vi "SwitchStateControl.vi"(5 "Switch Bit":bool=TRUE, 8 "error in (no error)":errorcluster, 9 "IP":string="172.16.7.43", 11 "Port":u16=9764) -> (0 "error out":errorcluster)   [LabVIEW 2009]
panel:
  in  "N Bit":u16=10
  in  "Register Number":u16=4
  out "Register read swapped":u32=1078
  out "Register swap":dbl[](array[numeric])=[0.0, 1.0, 1.0, 0.0, 1.0, 1.0, 0.0, 0.0, 0.0, 0.0, 1.0, 0.0, 0.0, 0.0, 0.0, 0.0, 0.0, 0.0, 0.0, 0.0, 0.0, 0.0, 0.0, 0.0, 0.0, 0.0, 0.0, 0.0, 0.0, 0.0, 0.0, 0.0]
  out "Register 4 bits":dbl[](array[numeric])=[0.0, 1.0, 1.0, 0.0, 1.0, 1.0, 0.0, 0.0, 0.0, 0.0, 1.0, 0.0, 0.0, 0.0, 0.0, 0.0, 0.0, 0.0, 0.0, 0.0, 0.0, 0.0, 0.0, 0.0, 0.0, 0.0, 0.0, 0.0, 0.0, 0.0, 0.0, 0.0]
  out "Register read":u32=1078
  in  "Device":u16(ring)=4 items=["Attenuation", "Clipping", "Enable channel", "Delay line", "ASIC"]
  # "SumMaj Bit\n        ll\n        v"
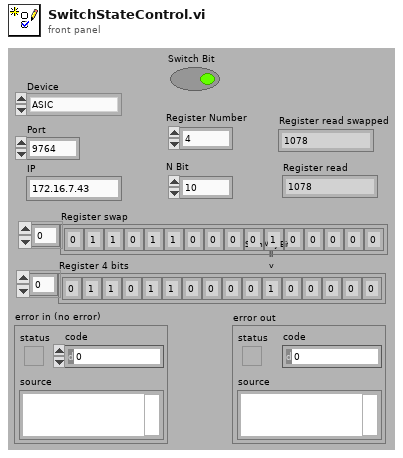
[diagram p1: front panel]
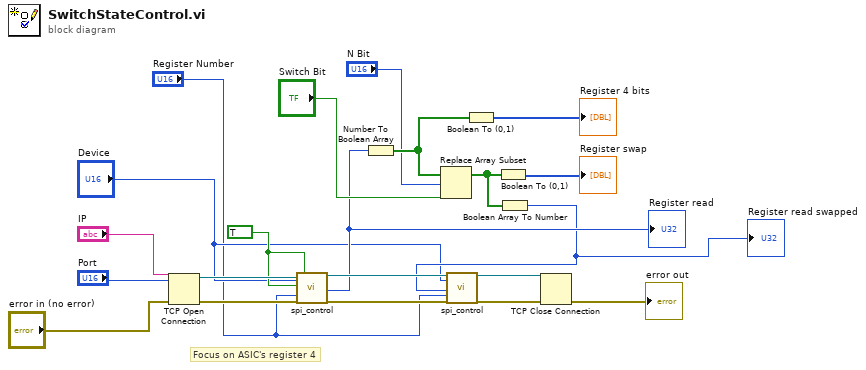
[diagram p0: block diagram]
diagram:
  w6 = TRUE
  # "Focus on ASIC's register 4"
  n1 = TCP Open Connection(address="IP", remote port or service name="Port", error in (no error)="error in (no error)") -> (connection ID=w18:refnum<k5>, error out=w19:errorcluster)  [unwired: 2 in]
  n2 = call "spi_control.vi"("connection ID"=w18, "Device"="Device", "Read/#write"=w6, "Register or channel"="Register Number", "error out 3"=w19, "Read physical"=w6) -> ("connection ID out"=w8:refnum<k5>, "data read value"=w5:u32, "error out 2"=w9:errorcluster)  [unwired: 6 in, 5 out]
  "Register read" <- w5
  n3 = Number To Boolean Array(number=w5) -> (Boolean array=w14:bool[])
  n4 = Replace Array Subset(array=w14, new element="Switch Bit", index="N Bit") -> (w11:bool[])
  n5 = Boolean To (0,1)(Boolean=w14) -> (0, 1=→"Register 4 bits":i16[])
  n6 = Boolean To (0,1)(Boolean=w11) -> (0, 1=→"Register swap":i16[])
  n7 = Boolean Array To Number(Boolean array=w11) -> (number=w4:u32)
  "Register read swapped" <- w4
  n8 = call "spi_control.vi"("connection ID"=w8, "Device"="Device", "Data"=w4, "Register or channel"="Register Number", "error out 3"=w9) -> ("connection ID out"=w7:refnum<k5>, "error out 2"=w10:errorcluster)  [unwired: 7 in, 6 out]
  n9 = TCP Close Connection(connection ID=w7, error in (no error)=w10) -> (error out=→"error out":errorcluster)  [unwired: 1 in, 1 out]
